vi "LEDExecute.vi"   [LabVIEW 2023]
uses:
  TheBox/BoxNoteState.ctl
  <vilib>/Rock Robotics/WPI/ThirdParty/PhotonVisionLib/PhotonVisionLib.lvlib
  <vilib>/Rock Robotics/WPI/DriverStation/WPI_DriverStationAllianceInfo.ctl
types:
  T1 = typedef "WPI_DriverStationAllianceInfo.ctl" = enum16{"Red", "Blue", "Invalid"}
  T2 = typedef "BoxNoteState.ctl" = enum16{"note in shooter wheels", "misaligned note", "no note", "have note"}
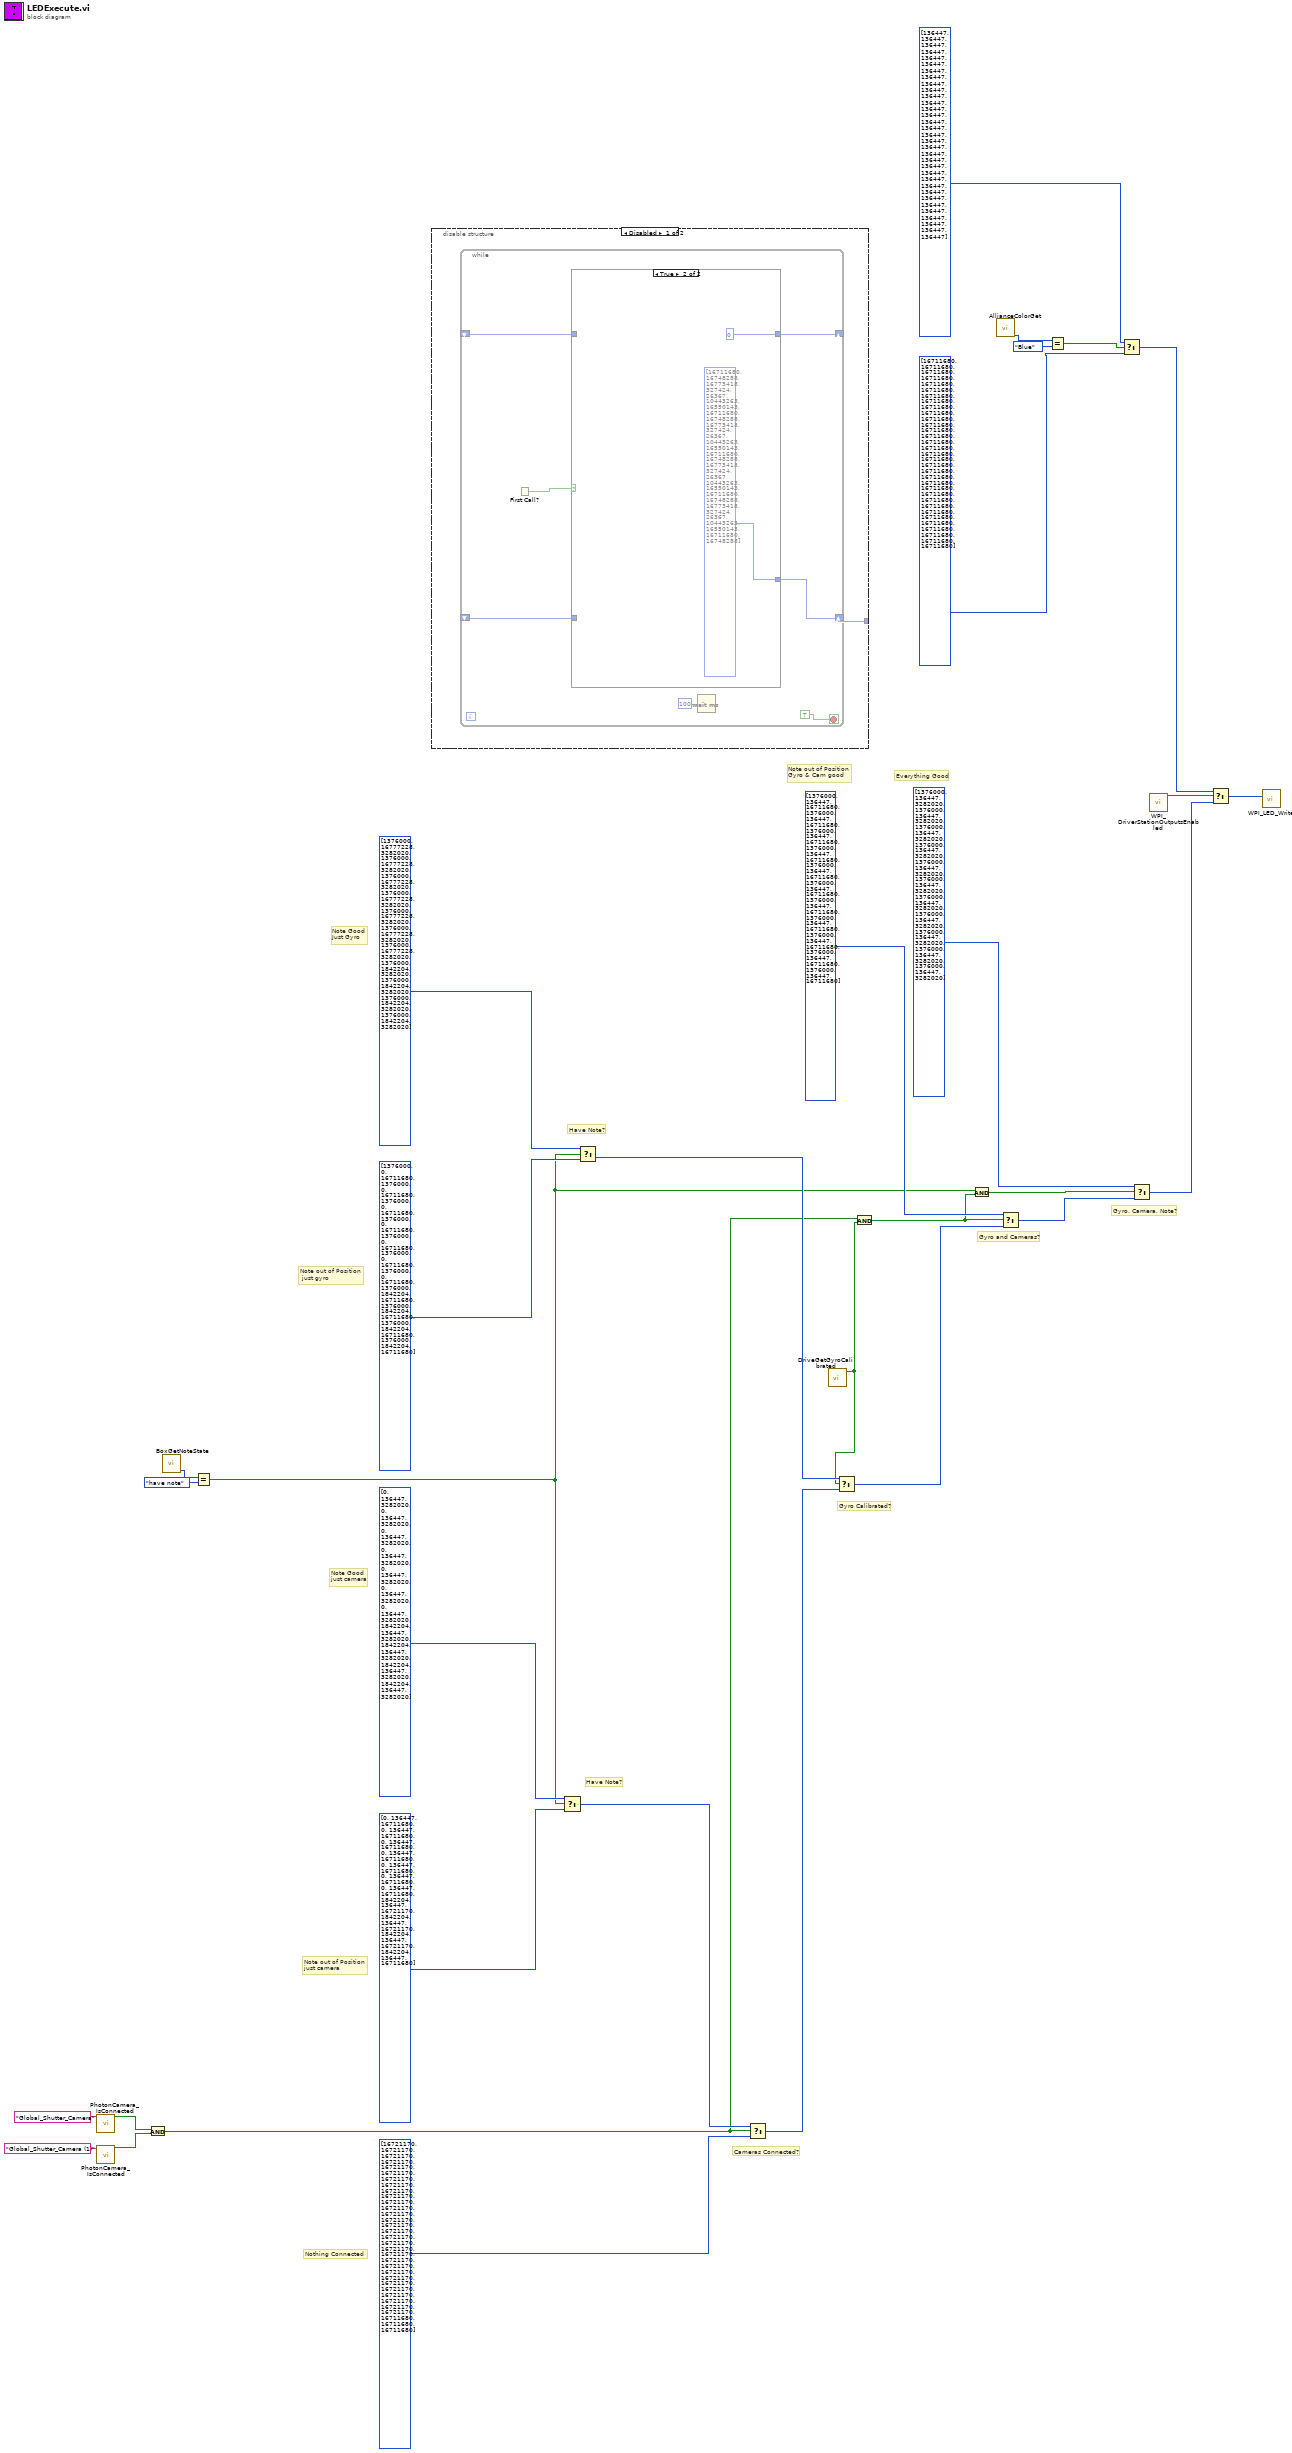
[diagram p0: block diagram]
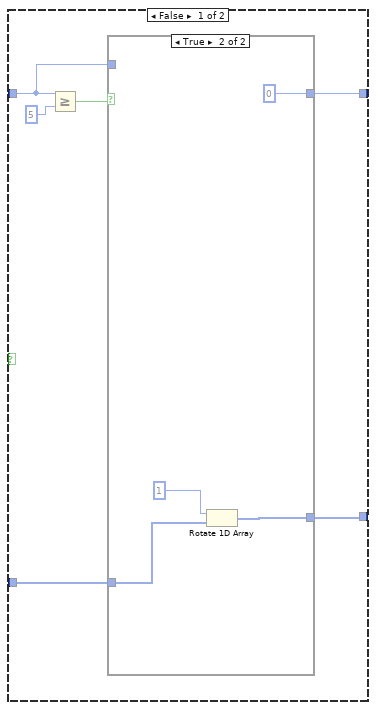
[diagram p2: hidden frame]
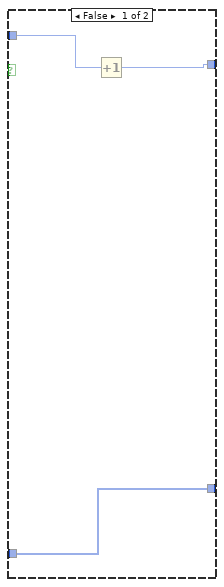
[diagram p3: hidden frame]
diagram:
  # "Gyro, Camera, Note?"
  # "Gyro and Cameras?"
  # "Gyro Calibrated?"
  # "Cameras Connected?"
  # "Have Note?"
  # "Have Note?"
  # "Note Good\njust camera"
  # "Note Good\nJust Gyro"
  # "Note out of Position\n just gyro"
  # "Note out of Position\njust camera"
  # "Everything Good"
  # "Note out of Position\nGyro & Cam good"
  # "Nothing Connected"
  n1 = call <vilib>:"PhotonCamera_IsConnected.vi"("CameraName"="Global_Shutter_Camera") -> ("IsConnected"=w9:bool)  [unwired: 9 in, 1 out]
  n2 = call <vilib>:"PhotonCamera_IsConnected.vi"("CameraName"="Global_Shutter_Camera (1)") -> ("IsConnected"=w8:bool)  [unwired: 9 in, 1 out]
  n3 = And(x=w9, y=w8) -> (x .and. y?=w12:bool)
  n4 = call "BoxGetNoteState.vi"() -> ("Box Note State"=w17:T2)  [unwired: 11 in]
  n5 = Equal?(x=w17, y=BoxNoteState."have note") -> (x = y?=w15:bool)
  n6 = disable-structure shown="Disabled" {
    disable-tunnel: [w33 _] -> _
    frame Disabled {
      n7 = while {
        shift-right: [w38] -> w33
        shift-left: _ -> [w35]
        shift-right: [w37] -> _
        shift-left: _ -> [w36]
        stop <- TRUE stop-if-true
        n8 = First Call?() -> (First Call?: T/F=w39:bool)
        n9 = case shown="True" w39 {
          tunnel: [w43 u32[] [16711680, 16748288, 16773418, 327424, 26367, 10443263, 16550143, 16711680, 16748288, 16773418, 327424, 26367, 10443263, 16550143, 16711680, 16748288, 16773418, 327424, 26367, 10443263, 16550143, 16711680, 16748288, 16773418, 327424, 26367, 10443263, 16550143, 16711680, 16748288] ("Color Array")] -> w38
          tunnel: [w42 0] -> w37
          tunnel: w36 -> [w41 _]
          tunnel: w35 -> [w44 _]
          frame False {
            n10 = Greater Or Equal?(x=w41, y=5) -> (x >= y?=w45:bool)
            n11 = case shown="True" w45 {
              tunnel: w44 -> [w47 w52]
              tunnel: [w47 w51] -> w43
              tunnel: [w49 0] -> w42
              tunnel: w41 -> [w48 _]
              frame False {
                n12 = Increment(x=w48) -> (x+1=w49:i32)
              }
              frame True {
                n13 = Rotate 1D Array(1:w52, 2:1 ("n")) -> (0:w51:u32[])
              }
            }
          }
          frame True {
          }
        }
        n14 = Wait (ms)(milliseconds to wait=u32 100) -> ()  [unwired: 1 out]
      }
    }
    frame Enabled {
    }
  }
  n15 = Select(t=u32[] [0, 136447, 3282020, 0, 136447, 3282020, 0, 136447, 3282020, 0, 136447, 3282020, 0, 136447, 3282020, 0, 136447, 3282020, 0, 136447, 3282020, 1842204, 136447, 3282020, 1842204, 136447, 3282020, 1842204, 136447, 3282020, 1842204, 136447, 3282020] ("Color Array"), s=w15, f=u32[] [0, 136447, 16711680, 0, 136447, 16711680, 0, 136447, 16711680, 0, 136447, 16711680, 0, 136447, 16711680, 0, 136447, 16711680, 0, 136447, 16711680, 1842204, 136447, 16721170, 1842204, 136447, 16721170, 1842204, 136447, 16721170, 1842204, 136447, 16711680] ("Color Array")) -> (s? t:f=w24:u32[])
  n16 = Select(t=u32[] [1376000, 16777228, 3282020, 1376000, 16777228, 3282020, 1376000, 16777228, 3282020, 1376000, 16777228, 3282020, 1376000, 16777228, 3282020, 1376000, 16777228, 3282020, 1376000, 16777228, 3282020, 1376000, 1842204, 3282020, 1376000, 1842204, 3282020, 1376000, 1842204, 3282020, 1376000, 1842204, 3282020] ("Color Array"), s=w15, f=u32[] [1376000, 0, 16711680, 1376000, 0, 16711680, 1376000, 0, 16711680, 1376000, 0, 16711680, 1376000, 0, 16711680, 1376000, 0, 16711680, 1376000, 0, 16711680, 1376000, 1842204, 16711680, 1376000, 1842204, 16711680, 1376000, 1842204, 16711680, 1376000, 1842204, 16711680] ("Color Array")) -> (s? t:f=w26:u32[])
  n17 = Select(t=w24, s=w12, f=u32[] [16721170, 16721170, 16721170, 16721170, 16721170, 16721170, 16721170, 16721170, 16721170, 16721170, 16721170, 16721170, 16721170, 16721170, 16721170, 16721170, 16721170, 16721170, 16721170, 16721170, 16721170, 16721170, 16721170, 16721170, 16721170, 16721170, 16721170, 16721170, 16721170, 16721170, 16711680, 16711680, 16711680] ("Color Array")) -> (s? t:f=w32:u32[])
  n18 = call "DriveGetGyroCalibrated.vi"() -> ("GryoCalibrated"=w7:bool)  [unwired: 11 in]
  n19 = Select(t=w26, s=w7, f=w32) -> (s? t:f=w30:u32[])
  n20 = And(x=w12, y=w7) -> (x .and. y?=w14:bool)
  n21 = And(x=w15, y=w14) -> (x .and. y?=w13:bool)
  n22 = call "AllianceColorGet.vi"() -> ("AllianceColor"=w6:T1)  [unwired: 11 in]
  n23 = Select(t=u32[] [1376000, 136447, 16711680, 1376000, 136447, 16711680, 1376000, 136447, 16711680, 1376000, 136447, 16711680, 1376000, 136447, 16711680, 1376000, 136447, 16711680, 1376000, 136447, 16711680, 1376000, 136447, 16711680, 1376000, 136447, 16711680, 1376000, 136447, 16711680, 1376000, 136447, 16711680] ("Color Array"), s=w14, f=w30) -> (s? t:f=w21:u32[])
  n24 = Equal?(x=w6, y=WPI_DriverStationAllianceInfo."Blue") -> (x = y?=w2:bool)
  n25 = Select(t=u32[] [136447, 136447, 136447, 136447, 136447, 136447, 136447, 136447, 136447, 136447, 136447, 136447, 136447, 136447, 136447, 136447, 136447, 136447, 136447, 136447, 136447, 136447, 136447, 136447, 136447, 136447, 136447, 136447, 136447, 136447, 136447, 136447, 136447] ("Color Array"), s=w2, f=u32[] [16711680, 16711680, 16711680, 16711680, 16711680, 16711680, 16711680, 16711680, 16711680, 16711680, 16711680, 16711680, 16711680, 16711680, 16711680, 16711680, 16711680, 16711680, 16711680, 16711680, 16711680, 16711680, 16711680, 16711680, 16711680, 16711680, 16711680, 16711680, 16711680, 16711680, 16711680, 16711680, 16711680] ("Color Array")) -> (s? t:f=w1:u32[])
  n26 = Select(t=u32[] [1376000, 136447, 3282020, 1376000, 136447, 3282020, 1376000, 136447, 3282020, 1376000, 136447, 3282020, 1376000, 136447, 3282020, 1376000, 136447, 3282020, 1376000, 136447, 3282020, 1376000, 136447, 3282020, 1376000, 136447, 3282020, 1376000, 136447, 3282020, 1376000, 136447, 3282020] ("Color Array"), s=w13, f=w21) -> (s? t:f=w20:u32[])
  n27 = call <vilib>:"WPI_DriverStationOutputsEnabled.vi"() -> ("OutputsEnabled?"=w29:bool)  [unwired: 10 in, 1 out]
  n28 = Select(t=w1, s=w29, f=w20) -> (s? t:f=w28:u32[])
  n29 = call <vilib>:"WPI_LED_Write.vi"("Color Array"=w28) -> ()  [unwired: 10 in, 1 out]
